vi "onStop.vi"(8 "error in (no error)":errorcluster, 11 "Server in":refnum<class "Server.lvclass">) -> (0 "error out":errorcluster, 3 "Server out":refnum<class "Server.lvclass">)   [LabVIEW 2013, in "MQTT Server.lvlib" / "Server.lvclass"]
uses:
  Server.lvclass
  MQTT_Base/MQTT_Base.lvclass
  Server.lvclass/Server.ctl
  ConnectionHandler/TCPConnectionHandler.lvclass
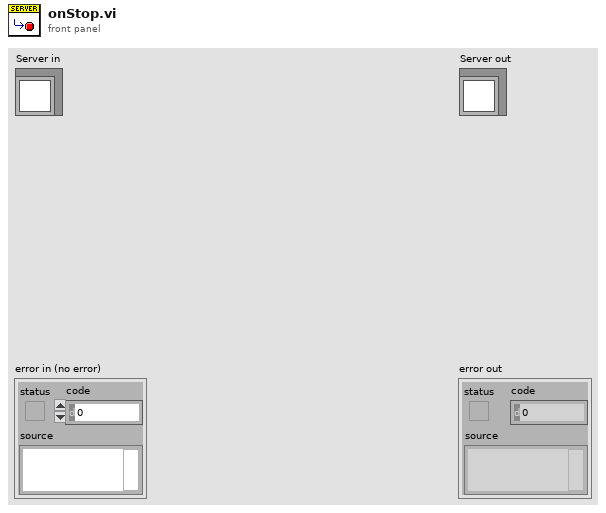
[diagram p1: front panel]
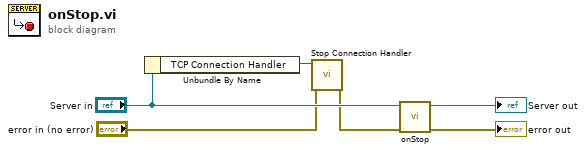
[diagram p0: block diagram]
diagram:
  n1 = Unbundle By Name("Server in") -> ("TCP Connection Handler"=w4:refnum<class "TCPConnectionHandler.lvclass">)
  n2 = call "Stop Connection Handler.vi"("error in (no error)"="error in (no error)", "TCPConnectionHandler in"=w4) -> ("error out"=w1:errorcluster)  [unwired: 8 in, 1 out]
  n3 = call-parent "onStop.vi"("error in (no error)"=w1, "MQTT_Base in"="Server in") -> ("error out"=→"error out":errorcluster, "MQTT_Base out"=→"Server out":refnum<class "Server.lvclass">)  [unwired: 8 in]
